vi "IS PolyVI Instance String to JSON Cluster.vi"(3 "Stream Time (optional)":timestamp=timestamp(1451714400 s since 1904-01-01), 4 "Stream Value":string, 5 "Stream Key":string) -> (1 "JSON Cluster Array out":T1[](array[typedef]))   [LabVIEW 2013]
uses:
  Custom Data Types/IS Data Point TypeDef (String).ctl
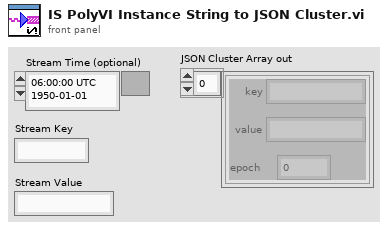
[diagram p1: front panel]
types:
  T1 = typedef "IS Data Point TypeDef (String).ctl" = cluster{"key":string, "value":string, "epoch":dbl}
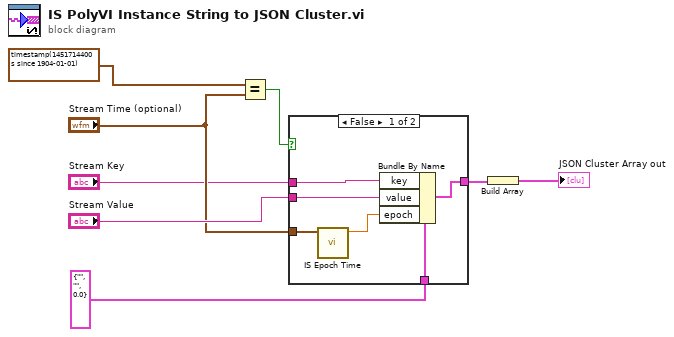
[diagram p0: block diagram]
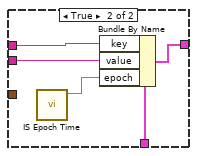
[diagram p2: hidden frame]
diagram:
  n1 = Equal?(x=timestamp(1451714400 s since 1904-01-01) ("Stream Time (optional)"), y="Stream Time (optional)") -> (x = y?=w2:bool)
  n2 = case shown="False" w2 {
    tunnel: T1 {"key"="", "value"="", "epoch"=0.0} ("IS Data point (String) 2") -> [w14 w19]
    tunnel: "Stream Key" -> [w13 w18]
    tunnel: [w11 w17] -> w7
    tunnel: "Stream Time (optional)" -> [w10 _]
    tunnel: "Stream Value" -> [w12 w15]
    frame False {
      n3 = call "IS Epoch Time.vi"("Stream Time (optional)"=w10) -> ("Time (epoch)"=w9:dbl)  [unwired: 10 in]
      n4 = Bundle By Name(cluster=w14, "key"=w13, "value"=w12, "epoch"=w9) -> (w11:T1)
    }
    frame True {
      n5 = call "IS Epoch Time.vi"() -> ("Time (epoch)"=w16:dbl)  [unwired: 11 in]
      n6 = Bundle By Name(cluster=w19, "key"=w18, "value"=w15, "epoch"=w16) -> (w17:T1)
    }
  }
  n7 = Build Array(w7) -> (→"JSON Cluster Array out":T1[])
